vi "subtract ref wavefront.vi"(8 "error in (no error)":errorcluster, 9 "HasoSlopes to output":refnum<class "HasoSlopes.lvclass">, 10 "Slopes file to subtract":path, 11 "HasoSlopes in":refnum<class "HasoSlopes.lvclass">) -> (0 "error out":errorcluster, 3 "HasoSlopes BG subtracted":refnum<class "HasoSlopes.lvclass">)   [LabVIEW 2020]
uses:
  WaveKit/Classes/HasoSlopes/HasoSlopes.lvclass
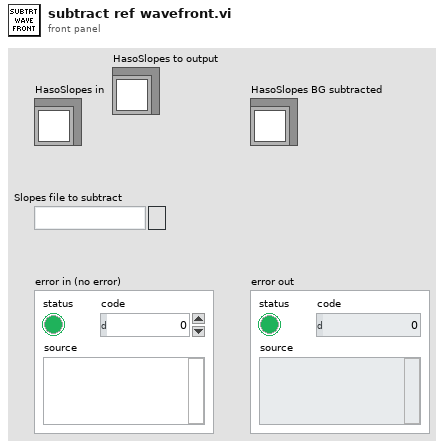
[diagram p1: front panel]
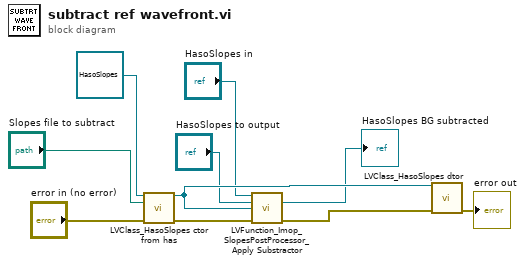
[diagram p0: block diagram]
diagram:
  n1 = call "LVClass_HasoSlopes ctor from has.vi"("HasoSlopes (const)"=refnum<class "HasoSlopes.lvclass"> refnum ("HasoSlopes in"), ".has path"="Slopes file to subtract", "error in (no error)"="error in (no error)") -> ("HasoSlopes (new)"=w10:refnum<class "HasoSlopes.lvclass">, "error out"=w6:errorcluster)  [unwired: 11 in]
  n2 = call "LVFunction_Imop_SlopesPostProcessor_Apply Substractor.vi"("HasoSlopes in"="HasoSlopes in", "HasoSlopes OUT"="HasoSlopes to output", "HasoSlopes to substract"=w10, "error in (no error)"=w6) -> ("HasoSlopes OUT 2"=→"HasoSlopes BG subtracted":refnum<class "HasoSlopes.lvclass">, "error out"=w7:errorcluster)  [unwired: 9 in, 1 out]
  n3 = call "LVClass_HasoSlopes dtor.vi"("HasoSlopes in"=w10, "error in (no error)"=w7) -> ("error out"=→"error out":errorcluster)  [unwired: 12 in, 1 out]
